vi "Word Report.vi"(0 "标题配置":cluster{"title":string, "font":T2}={"title"="测试报告", "font"={"font name"="", "font size"=24.0, "bold"=2, "italic"=2, "underline"=2, "strike through"=2, "font color"=16777222}} {"font"."font size" format="%0.2f"; "font"."strike through" items=["Unchanged", "Yes", "No"]; "font"."underline" items=["Unchanged", "Yes", "No"]; "font"."italic" items=["Unchanged", "Yes", "No"]; "font"."bold" items=["Unchanged", "Yes", "No"]}, 1 "测试信息":cluster{"font":T2, "字符串":string}={"font"={"font name"="", "font size"=12.0, "bold"=2, "italic"=2, "underline"=2, "strike through"=2, "font color"=16777222}, "字符串"="1"} {"font"."font size" format="%0.2f"; "font"."strike through" items=["Strk Unchanged", "Strk Yes", "Strk No"]; "font"."underline" items=["Und Unchanged", "Und Yes", "Und No"]; "font"."italic" items=["Ital Unchanged", "Ital Yes", "Ital No"]; "font"."bold" items=["Bold Unchanged", "Bold Yes", "Bold No"]}, 2 "文本":cluster{"font":T2, "字符串":string}={"font"={"font name"="", "font size"=12.0, "bold"=2, "italic"=2, "underline"=2, "strike through"=2, "font color"=16777222}, "字符串"="2"} {"font"."font size" format="%0.2f"; "font"."strike through" items=["Strk Unchanged", "Strk Yes", "Strk No"]; "font"."underline" items=["Und Unchanged", "Und Yes", "Und No"]; "font"."italic" items=["Ital Unchanged", "Ital Yes", "Ital No"]; "font"."bold" items=["Bold Unchanged", "Bold Yes", "Bold No"]}, 3 "表格":T3={"auto format"=11, "font"={"font name"="", "font size"=0.0, "bold"=0, "italic"=0, "underline"=0, "strike through"=0, "font color"=0}, "表格 2"=[["1", "1.5", "5.6", "5.6", "7.9", "4.6"], ["2", "2.5", "7.6", "6.5", "7.2", "7.5"], ["3", "6.8", "9.1", "4.2", "6.2", "6.1"], ["4", "6.7", "7.1", "7.2", "1.0", "8.3"], ["5", "6.4", "4.3", "9.2", "5.8", "4.2"], ["6", "8.6", "8.2", "4.3", "8.6", "4.5"]]} {"auto format" items=["xlRangeAutoFormat3DEffects1"=13, "xlRangeAutoFormat3DEffects2"=14, "xlRangeAutoFormatAccounting1"=4, "xlRangeAutoFormatAccounting2"=5, "xlRangeAutoFormatAccounting3"=6, "xlRangeAutoFormatAccounting4"=17, "xlRangeAutoFormatClassic1"=1, "xlRangeAutoFormatClassic2"=2, "xlRangeAutoFormatClassic3"=3, "xlRangeAutoFormatColor1"=7, "xlRangeAutoFormatColor2"=8, "xlRangeAutoFormatColor3"=9, "xlRangeAutoFormatList1"=10, "xlRangeAutoFormatList2"=11, "xlRangeAutoFormatList3"=12, "xlRangeAutoFormatLocalFormat1"=15, "xlRangeAutoFormatLocalFormat2"=16, "xlRangeAutoFormatLocalFormat3"=19, "xlRangeAutoFormatLocalFormat4"=20, "xlRangeAutoFormatReport1"=21, "xlRangeAutoFormatReport2"=22, "xlRangeAutoFormatReport3"=23, "xlRangeAutoFormatReport4"=24, "xlRangeAutoFormatReport5"=25, "xlRangeAutoFormatReport6"=26, "xlRangeAutoFormatReport7"=27, "xlRangeAutoFormatReport8"=28, "xlRangeAutoFormatReport9"=29, "xlRangeAutoFormatReport10"=30, "xlRangeAutoFormatClassicPivotTable"=31, "xlRangeAutoFormatTable1"=32, "xlRangeAutoFormatTable2"=33, "xlRangeAutoFormatTable3"=34, "xlRangeAutoFormatTable4"=35, "xlRangeAutoFormatTable5"=36, "xlRangeAutoFormatTable6"=37, "xlRangeAutoFormatTable7"=38, "xlRangeAutoFormatTable8"=39, "xlRangeAutoFormatTable9"=40, "xlRangeAutoFormatTable10"=41, "xlRangeAutoFormatPTNone"=42, "xlRangeAutoFormatNone"=-4142, "xlRangeAutoFormatSimple"=-4154]; "font"."font size" format="%0.2f"; "font"."strike through" items=["Strk Unchanged", "Strk Yes", "Strk No"]; "font"."underline" items=["Und Unchanged", "Und Yes", "Und No"]; "font"."italic" items=["Ital Unchanged", "Ital Yes", "Ital No"]; "font"."bold" items=["Bold Unchanged", "Bold Yes", "Bold No"]}, 4 "图表配置":T4={"chart type"=4, "graph title (\"\")"="测试图表"} {"chart type" items=["xlColumnClustered"=51, "xlColumnStacked"=52, "xlColumnStacked100"=53, "xl3DColumnClustered"=54, "xl3DColumnStacked"=55, "xl3DColumnStacked100"=56, "xlBarClustered"=57, "xlBarStacked"=58, "xlBarStacked100"=59, "xl3DBarClustered"=60, "xl3DBarStacked"=61, "xl3DBarStacked100"=62, "xlLineStacked"=63, "xlLineStacked100"=64, "xlLineMarkers"=65, "xlLineMarkersStacked"=66, "xlLineMarkersStacked100"=67, "xlPieOfPie"=68, "xlPieExploded"=69, "xl3DPieExploded"=70, "xlBarOfPie"=71, "xlXYScatterSmooth"=72, "xlXYScatterSmoothNoMarkers"=73, "xlXYScatterLines"=74, "xlXYScatterLinesNoMarkers"=75, "xlAreaStacked"=76, "xlAreaStacked100"=77, "xl3DAreaStacked"=78, "xl3DAreaStacked100"=79, "xlDoughnutExploded"=80, "xlRadarMarkers"=81, "xlRadarFilled"=82, "xlSurface"=83, "xlSurfaceWireframe"=84, "xlSurfaceTopView"=85, "xlSurfaceTopViewWireframe"=86, "xlBubble"=15, "xlBubble3DEffect"=87, "xlStockHLC"=88, "xlStockOHLC"=89, "xlStockVHLC"=90, "xlStockVOHLC"=91, "xlCylinderColClustered"=92, "xlCylinderColStacked"=93, "xlCylinderColStacked100"=94, "xlCylinderBarClustered"=95, "xlCylinderBarStacked"=96, "xlCylinderBarStacked100"=97, "xlCylinderCol"=98, "xlConeColClustered"=99, "xlConeColStacked"=100, "xlConeColStacked100"=101, "xlConeBarClustered"=102, "xlConeBarStacked"=103, "xlConeBarStacked100"=104, "xlConeCol"=105, "xlPyramidColClustered"=106, "xlPyramidColStacked"=107, "xlPyramidColStacked100"=108, "xlPyramidBarClustered"=109, "xlPyramidBarStacked"=110, "xlPyramidBarStacked100"=111, "xlPyramidCol"=112, "xl3DColumn"=-4100, "xlLine"=4, "xl3DLine"=-4101, "xl3DPie"=-4102, "xlPie"=5, "xlXYScatter"=-4169, "xl3DArea"=-4098, "xlArea"=1, "xlDoughnut"=-4120, "xlRadar"=-4151]}, 6 "报告类型":u16(ring)=1, 7 "簇":T1={"Save Report 2"=FALSE, "路径"=path "/Report.html", "Print Report 2"=FALSE, "份数"=1} {"份数" min=1 max=10 step=1}) -> ()   [LabVIEW 2014]
uses:
  <vilib>/addons/_office/_wordsub.llb/font.ctl
  <vilib>/addons/_office/word.llb/Word Easy Table (str).vi
  <vilib>/Utility/NIReport.llb/NI_report.lvclass
  <vilib>/Utility/NIReport.llb/Word/NI_Word.lvclass
  <vilib>/addons/_office/NI_ReportGenerationToolkit.lvlib
panel:
  out "表格 2":string[][](table)=[["1", "1.5", "5.6", "5.6", "7.9", "4.6"], ["2", "2.5", "7.6", "6.5", "7.2", "7.5"], ["3", "6.8", "9.1", "4.2", "6.2", "6.1"], ["4", "6.7", "7.1", "7.2", "1.0", "8.3"], ["5", "6.4", "4.3", "9.2", "5.8", "4.2"], ["6", "8.6", "8.2", "4.3", "8.6", "4.5"]]
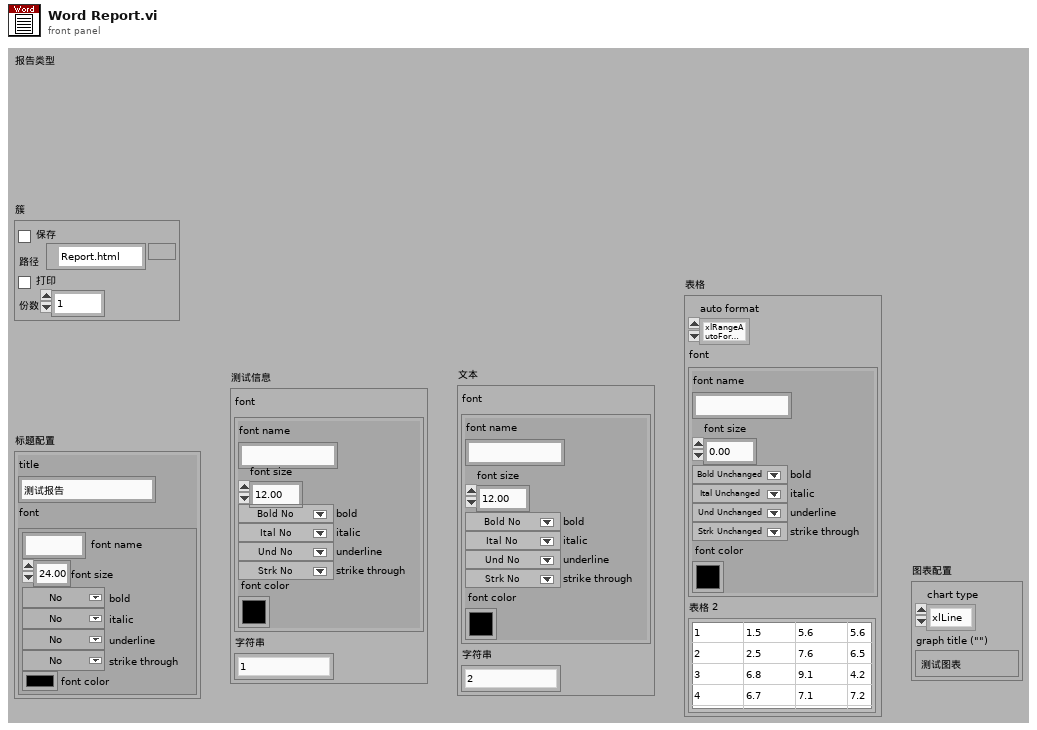
[diagram p1: front panel]
types:
  T1 = cluster{"Save Report 2":bool, "路径":path, "Print Report 2":bool, "份数":i32}
  T2 = typedef "font.ctl" = cluster{"font name":string, "font size":dbl, "bold":u16, "italic":u16, "underline":u16, "strike through":u16, "font color":u32}
  T3 = cluster{"auto format":i32, "font":T2, "表格 2":string[][]}
  T4 = cluster{"chart type":i32, "graph title (\"\")":string}
  T5 = typedef "Generate Report Object Reference.ctl" = refnum<class "NI_report.lvclass">
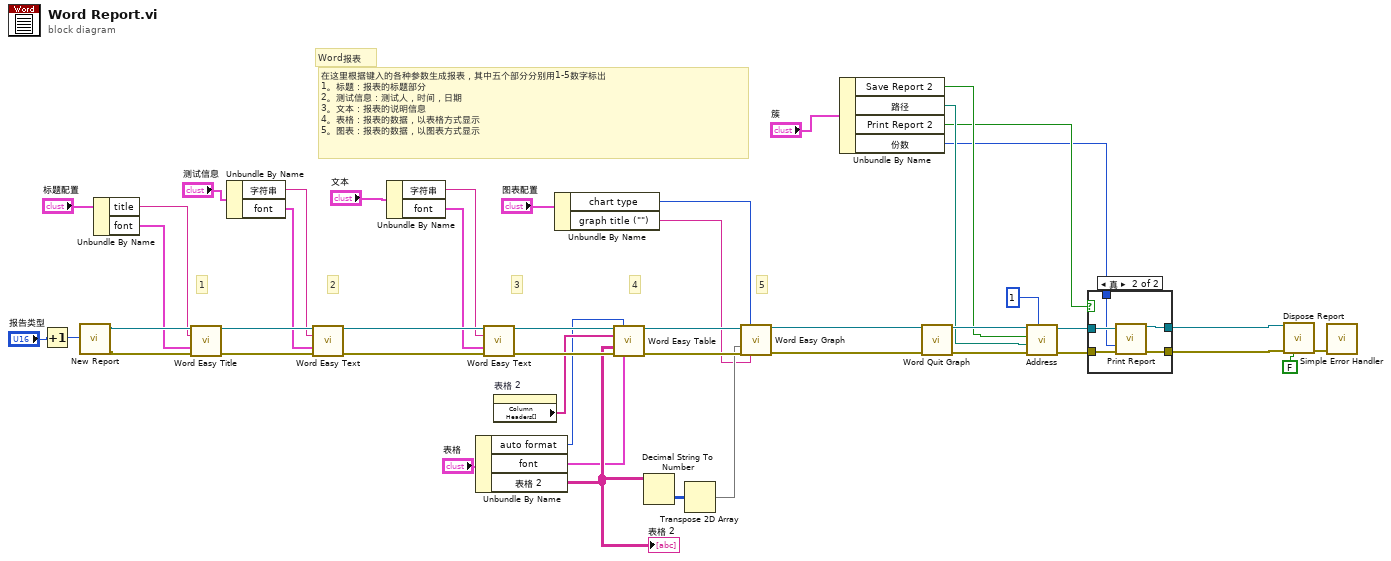
[diagram p0: block diagram]
diagram:
  # "3"
  # "2"
  # "Word报表"
  # "5"
  # "4"
  # "1"
  # "在这里根据键入的各种参数生成报表，其中五个部分分别用1-5数字标出\n1。标题：报表的标题部分\n2。测试信息：测试人，时间，日期\n3。文本：报表的说明信息\n4。表格：报表的数据，以表格方式显示\n5。图表：报表的数据，以图表方式显示"
  n1 = Increment(x="报告类型") -> (x+1=w41:u16)
  n2 = call <vilib>:"New Report.vi"("report type"=w41) -> ("report out"=w22:refnum<class "NI_report.lvclass">, "error out"=w21:errorcluster)  [unwired: 13 in]
  n3 = Unbundle By Name("标题配置") -> ("title"=w20:string, "font"=w19:T2)
  n4 = call <vilib>:"Word Easy Title.vi"("report in"=w22, "title"=w20, "font"=w19, "error in (no error)"=w21) -> ("report out"=w36:refnum<class "NI_report.lvclass">, "error out"=w35:errorcluster)  [unwired: 9 in, 1 out]
  n5 = Unbundle By Name("测试信息") -> ("字符串"=w17:string, "font"=w18:T2)
  n6 = call <vilib>:"Word Easy Text.vi"("report in"=w36, "text"=w17, "font"=w18, "error in (no error)"=w35) -> ("report out"=w33:refnum<class "NI_report.lvclass">, "error out"=w32:errorcluster)  [unwired: 9 in, 1 out]
  n7 = Unbundle By Name("文本") -> ("字符串"=w16:string, "font"=w15:T2)
  n8 = Unbundle By Name("表格") -> ("auto format"=w1:i32, "font"=w2:T2, "表格 2"=w12:string[][])
  "表格 2" <- w12
  n9 = call <vilib>:"Word Easy Text.vi"("report in"=w33, "text"=w16, "font"=w15, "error in (no error)"=w32) -> ("report out"=w34:refnum<class "NI_report.lvclass">, "error out"=w14:errorcluster)  [unwired: 9 in, 1 out]
  n10 = property on="表格 2" class="Tbl (严格)"() -> ("Column Headers[]"=w13:string[])  [unwired: 2 in, 2 out]
  n11 = Unbundle By Name("图表配置") -> ("chart type"=w9:i32, "graph title (\"\")"=w10:string)
  n12 = call-poly <vilib>:"Word Easy Table.vi"("report in"=w34, "auto format (none)"=w1, "row headers"=w13, "data"=w12, "error in (no error)"=w14, "font"=w2) -> ("report out"=w38:refnum<class "NI_report.lvclass">, "error out"=w37:errorcluster)  [unwired: 7 in, 1 out]
  n13 = Decimal String To Number(string=w12) -> (number=w42:i32[][])  [unwired: 2 in, 1 out]
  n14 = Transpose 2D Array(2D array=w42) -> (transposed array=w11:i32[][])
  n15 = call <vilib>:"Word Easy Graph.vi"("report in"=w38, "graph type (col clustered)"=w9, "data"=w11, "error in (no error)"=w37, "graph title (\"\")"=w10) -> ("report out"=w8:refnum<class "NI_report.lvclass">, "error out"=w7:errorcluster)  [unwired: 9 in]
  n16 = Unbundle By Name("簇") -> ("Save Report 2"=w6:bool, "路径"=w5:path, "Print Report 2"=w4:bool, "份数"=w3:i32)
  n17 = call <vilib>:"Word Quit Graph.vi"("report in"=w8, "error in (no error)"=w7) -> ("report out"=w27:refnum<class "NI_report.lvclass">, "error out"=w26:errorcluster)  [unwired: 12 in]
  n18 = call "Address.vi"("报告类型"=u16 1 ("报告类型 2"), "错误簇输入"=w26, "路径"=w5, "保存？"=w6, "报告输入"=w27) -> ("错误簇输出"=w24:errorcluster, "报告输出"=w25:T5)  [unwired: 5 in]
  n19 = case shown="真" w4 {
    tunnel: w24 -> [w48 w52]
    tunnel: w25 -> [w49 w51]
    tunnel: [w49 w53] -> w29
    tunnel: [w48 w54] -> w31
    tunnel: w3 -> [_ w50]
    frame False {
    }
    frame True {
      n20 = call-dynamic "Print Report.vi"("report in"=w51, "number of copies (1)"=w50, "error in (no error)"=w52) -> ("report out"=w53:T5, "error out"=w54:errorcluster)  [unwired: 11 in]
    }
  }
  n21 = call-dynamic "Dispose Report.vi"("report in"=w29, "error in (no error)"=w31, "close report? (T)"=FALSE ("Close Report? (T)")) -> ("error out"=w30:errorcluster)  [unwired: 12 in]
  n22 = call <vilib>:"Simple Error Handler.vi"("error in (no error)"=w30) -> ()  [unwired: 4 in, 5 out]
